vi "Parse Signal List.vi"(8 "error in":errorcluster, 11 "MLTFNC in":refnum<class "MLTFNC.lvclass">) -> (0 "error out":errorcluster, 3 "MLTFNC out":refnum<class "MLTFNC.lvclass">)   [LabVIEW 2019, in "MLTFNC.lvlib" / "MLTFNC.lvclass"]
uses:
  Library/MLTFNC.lvclass
  C:/Users/Public/Documents/Development/builds/Tools/Config.lvlibp/Config.lvclass
  Library/MLTFNC.lvclass/MLTFNC.ctl
  builds/Tools/Config.lvlibp/Accessors/Read Device Signals.vi
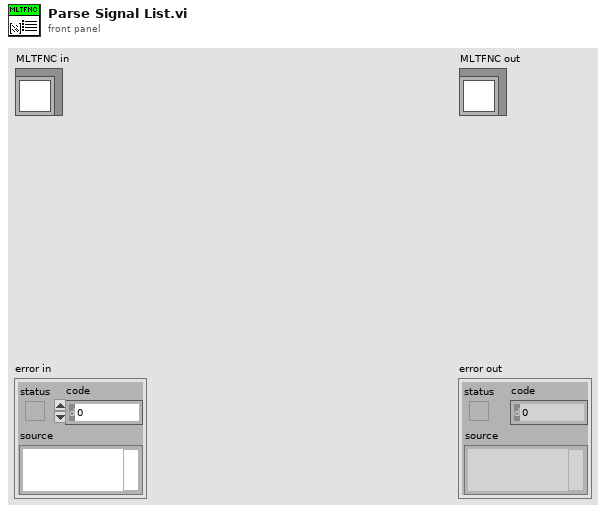
[diagram p1: front panel]
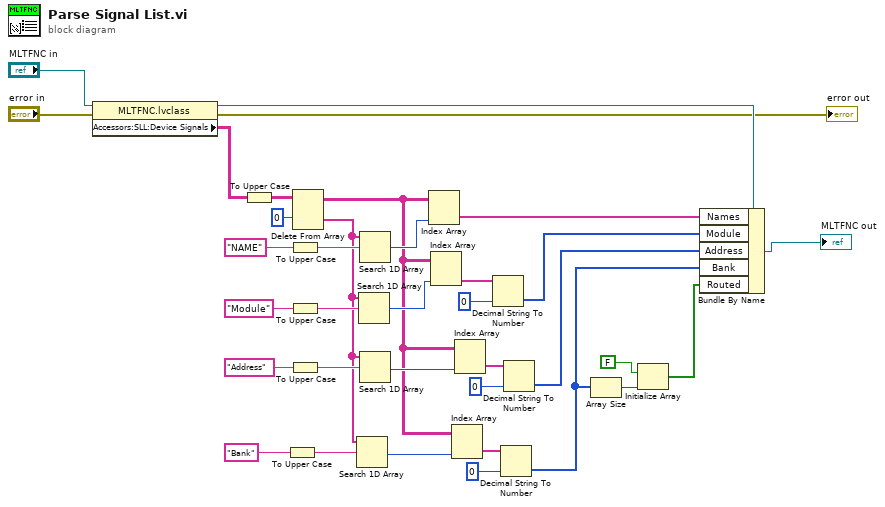
[diagram p0: block diagram]
diagram:
  n1 = property class="MLTFNC.lvclass"(reference="MLTFNC in", error in="error in") -> (reference out=w33:refnum<class "MLTFNC.lvclass">, error out=→"error out":errorcluster, "Accessors:SLL:Device Signals"=w32:string[][])
  n2 = To Upper Case(1:w32) -> (0:w23:string[][])
  n3 = To Upper Case(1:"Bank" ("element")) -> (0:w11:string)
  n4 = To Upper Case(1:"NAME" ("element")) -> (0:w18:string)
  n5 = To Upper Case(1:"Module" ("element")) -> (0:w17:string)
  n6 = To Upper Case(1:"Address" ("element")) -> (0:w16:string)
  n7 = Delete From Array(array=w23, index (row)=0) -> (deleted portion=w5:string[], array with subset deleted=w8:string[][])  [unwired: 2 in]
  n8 = Search 1D Array(1D array=w5, element=w11) -> (index of element=w9:i32)  [unwired: 1 in]
  n9 = Search 1D Array(1D array=w5, element=w17) -> (index of element=w24:i32)  [unwired: 1 in]
  n10 = Search 1D Array(1D array=w5, element=w18) -> (index of element=w30:i32)  [unwired: 1 in]
  n11 = Search 1D Array(1D array=w5, element=w16) -> (index of element=w20:i32)  [unwired: 1 in]
  n12 = Index Array(array=w8, index (col)=w30) -> (element=w28:string[])  [unwired: 1 in]
  n13 = Index Array(array=w8, index (col)=w24) -> (element=w27:string[])  [unwired: 1 in]
  n14 = Index Array(array=w8, index (col)=w9) -> (element=w13:string[])  [unwired: 1 in]
  n15 = Index Array(array=w8, index (col)=w20) -> (element=w14:string[])  [unwired: 1 in]
  n16 = Decimal String To Number(string=w27, default (0L)=u32 0 ("Numeric")) -> (number=w7:u32[])  [unwired: 1 in, 1 out]
  n17 = Decimal String To Number(string=w13, default (0L)=u32 0 ("Numeric")) -> (number=w4:u32[])  [unwired: 1 in, 1 out]
  n18 = Decimal String To Number(string=w14, default (0L)=u32 0 ("Numeric")) -> (number=w6:u32[])  [unwired: 1 in, 1 out]
  n19 = Array Size(array=w4) -> (size(s)=w3:i32)
  n20 = Initialize Array(FALSE, w3) -> (w1:bool[])
  n21 = Bundle By Name(cluster=w33, "Names"=w28, "Module"=w7, "Address"=w6, "Bank"=w4, "Routed"=w1) -> (→"MLTFNC out":refnum<class "MLTFNC.lvclass">)
